vi "GEvt-Generate Register Log.vi"(0 "CSM Global Log Event":refnum<user-event>, 1 "Current State":string, 2 "Arguments":string, 6 "Name(\"\" to use uuid)":string, 10 "CSM:LogFilter.lvclass":refnum<class "LogFilter.lvclass">) -> (14 "CSM Global Log Event out":refnum<user-event>, 16 "event data":T1={"Name(\"\" to use uuid)"="", "Current State"="", "Arguments"="", "Source Message"={"‘State"="", "’Arguments"="", "’Error"={"status"=FALSE, "code"=0, "source"=""}}, "Source Module"="", "Complete(T)/Start(F)"=FALSE, "LogType"=enum."State Change"})   [LabVIEW 2020, in "Communicable State Machine.lvlib"]
uses:
  Communicable State Machine.lvlib
  _CSM_GlobalLog_MSG.ctl
  _CSM_Response Source Message.ctl
  _CSM_GlobalLog_MSG_TYPE.ctl
  LogFilter.lvclass
  Filter Check.vi
  Group Check - CSM.vi
  Group Check - LogType.vi
  Group Check - State.vi
  CSM Check - LogType.vi
  CSM Check - State.vi
  CSM Check - StateType.vi
  Group Check - StateType.vi
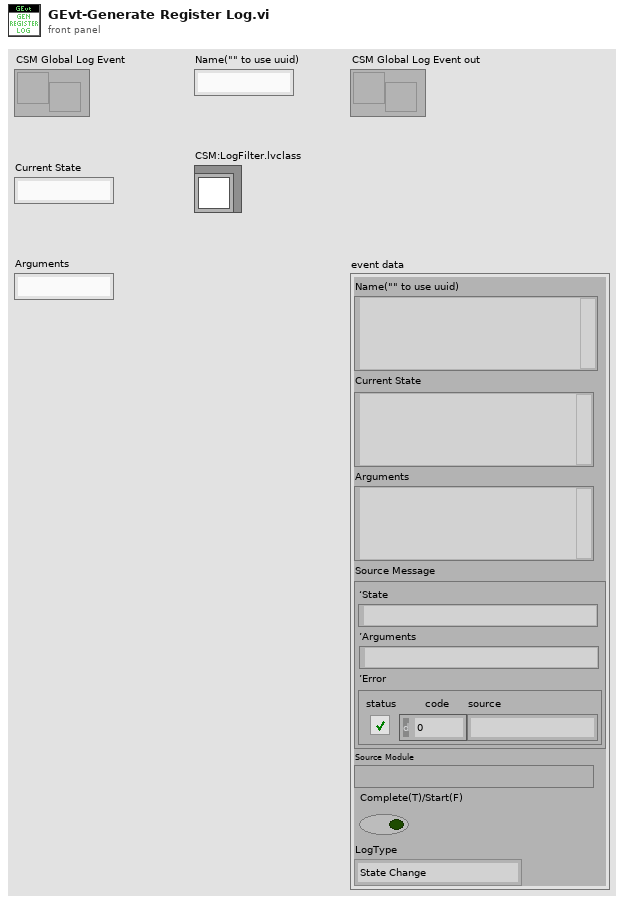
[diagram p1: front panel]
types:
  T1 = typedef "Communicable State Machine.lvlib/_CSM_GlobalLog_MSG.ctl" = cluster{"Name(\"\" to use uuid)":string, "Current State":string, "Arguments":string, "Source Message":T2, "Source Module":string, "Complete(T)/Start(F)":bool, "LogType":T3}
  T2 = typedef "Communicable State Machine.lvlib/_CSM_Response Source Message.ctl" = cluster{"‘State":string, "’Arguments":string, "’Error":errorcluster}
  T3 = typedef "Communicable State Machine.lvlib/_CSM_GlobalLog_MSG_TYPE.ctl" = enum16{"User Log", "State Change", "Status", "Interrupt", "Register", "Unregister", "Error Log", "Module Created", "Module Destroyed"}
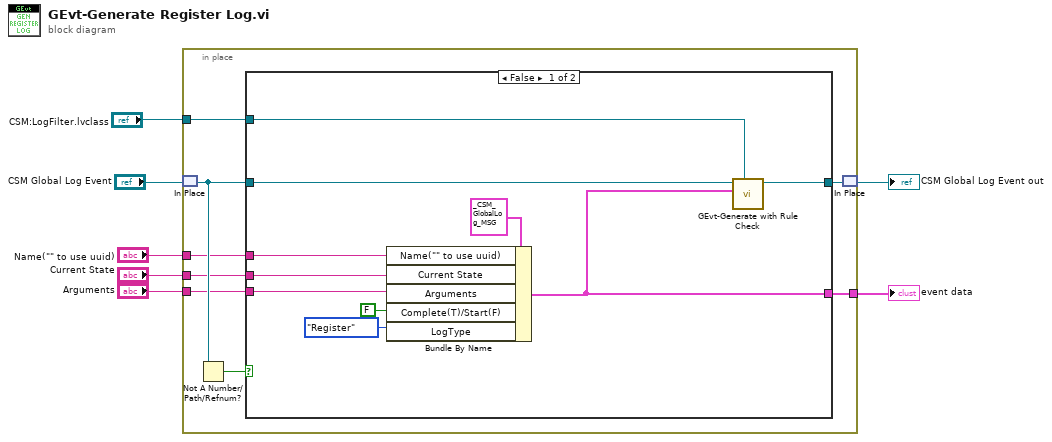
[diagram p0: block diagram]
diagram:
  n1 = in-place {
    in-place-border: [w12] -> w5
    in-place-border: "Name(\"\" to use uuid)" -> [w11]
    in-place-border: "Current State" -> [w10]
    in-place-border: "Arguments" -> [w9]
    in-place-border: "CSM:LogFilter.lvclass" -> [w8]
    n2 = in-place-match #1("CSM Global Log Event") -> (w14:refnum<user-event>)
    n3 = Not A Number/Path/Refnum?(number/path/refnum=w14) -> (NaN/Path/Refnum?=w15:bool)
    n4 = case shown="False" w15 {
      tunnel: w14 -> [w25 w26]
      tunnel: [w24 w26] -> w13
      tunnel: [w16 _] -> w12
      tunnel: w11 -> [w20 _]
      tunnel: w10 -> [w19 _]
      tunnel: w9 -> [w18 _]
      tunnel: w8 -> [w17 _]
      frame False {
        n5 = Bundle By Name(cluster=T1 {"Name(\"\" to use uuid)"="", "Current State"="", "Arguments"="", "Source Message"={"‘State"="", "’Arguments"="", "’Error"={"status"=FALSE, "code"=0, "source"=""}}, "Source Module"="", "Complete(T)/Start(F)"=FALSE, "LogType"=enum."State Change"} ("event data"), "Name(\"\" to use uuid)"=w20, "Current State"=w19, "Arguments"=w18, "Complete(T)/Start(F)"=FALSE, "LogType"=_CSM_GlobalLog_MSG_TYPE."Register" ("Type")) -> (w16:T1)
        n6 = call "GEvt-Generate with Rule Check.vi"("LogFilter in"=w17, "event data"=w16, "CSM Global Log Event in"=w25) -> ("CSM Global Log Event out"=w24:refnum<user-event>)  [unwired: 8 in]
      }
      frame True {
      }
    }
    n7 = in-place-match #1(w13) -> (→"CSM Global Log Event out":refnum<user-event>)
  }
  "event data" <- w5
